vi "ROS_Publisher.vi"() -> ()   [LabVIEW 2016]
doc: "The ROS publisher bundles together several variables into a \"MasterMessage\" that is published on the ROS network. If there is an error in the ROS Write node the VI is exited."
uses:
  <userlib>/ROS for LabVIEW Software/ROS/Code/Console/Servers/ServerSubs/TopicDef.ctl
  <userlib>/ROS for LabVIEW Software/ROS/Code/SubVIs/_ROSDirection.ctl
  GlobalVI.vi
  <userlib>/ROS for LabVIEW Software/ROS/Code/_ROSDefinition.vi
panel:
  out "ROS Write ERR":errorcluster
  out "JSON string 2":string
  out "error out":errorcluster
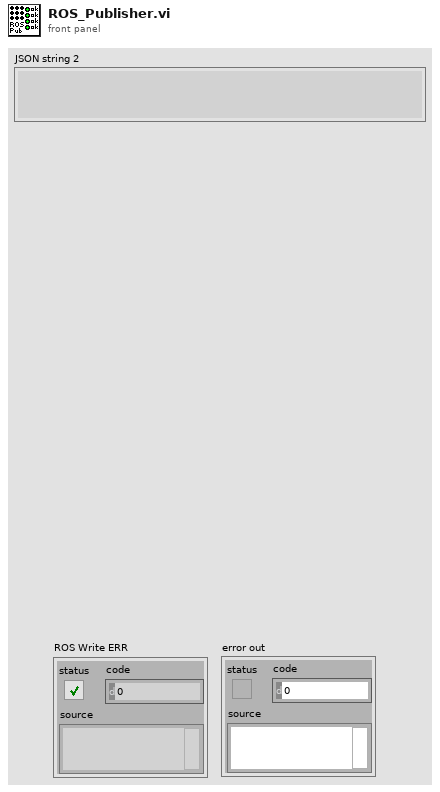
[diagram p1: front panel]
types:
  T1 = typedef "TopicDef.ctl" = cluster{"Topic":string, "Type":string, "Action":T2, "Update (ms)":u16, "queue size":u16}
  T2 = typedef "_ROSDirection.ctl" = enum16{"Node", "Publisher", "Subscriber", "ServiceClient", "ServiceProvider"}
  T3 = typedef "_ROSControl.ctl" = cluster{"topic port":u16, "Node":string, "topic":string, "type":string, "node port":u16, "error ":errorcluster, "Direction":T2, "Update (ms)":u16, "FIFO size":u16}
  T4 = cluster{"status":cluster{"liftStatus":bool, "lidarBackStatus":bool, "uwbStatus":bool, "lightStatus":bool}}
  T5 = cluster{"liftStatus":bool, "lidarBackStatus":bool, "uwbStatus":bool, "lightStatus":bool}
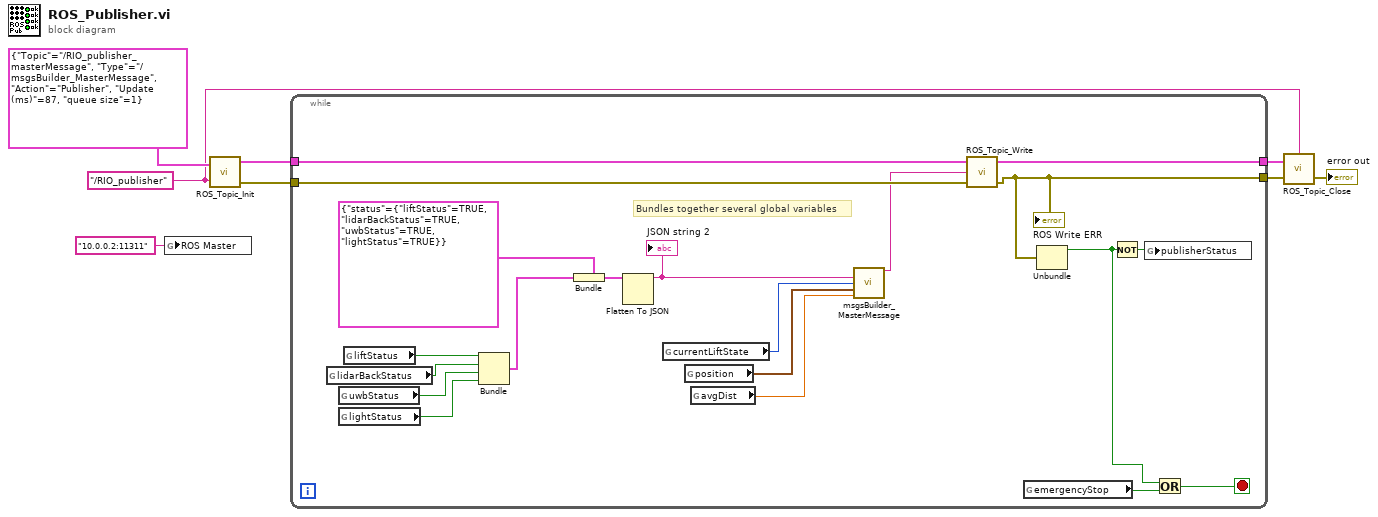
[diagram p0: block diagram]
diagram:
  w7 = "/RIO_publisher" ("node")
  n1 = global write "_ROSDefinition.vi" "ROS Master"("10.0.0.2:11311" ("ROS Master")) -> ()
  n2 = call <userlib>:"ROS_Topic_Init.vi"("Definitions"=T1 {"Topic"="/RIO_publisher_masterMessage", "Type"="/msgsBuilder_MasterMessage", "Action"=enum."Publisher", "Update (ms)"=87, "queue size"=1}, "node"=w7) -> ("ROS out"=w6:T3, "error out"=w1:errorcluster)  [unwired: 1 in]
  n3 = while {
    tunnel: w6 -> [w28]
    tunnel: [w27] -> w5
    tunnel: w1 -> [w26]
    tunnel: [w18] -> w4
    stop <- w16 stop-if-true
    # "Bundles together several global variables"
    n4 = global read "GlobalVI.vi" "lidarBackStatus"() -> (w23:bool)
    n5 = global read "GlobalVI.vi" "uwbStatus"() -> (w24:bool)
    n6 = global read "GlobalVI.vi" "lightStatus"() -> (w25:bool)
    n7 = global read "GlobalVI.vi" "liftStatus"() -> (w22:bool)
    n8 = Bundle("liftStatus"=w22, "lidarBackStatus"=w23, "uwbStatus"=w24, "lightStatus"=w25) -> (w20:T5)  [unwired: 1 in]
    n9 = Bundle(cluster=T4 {"status"={"liftStatus"=TRUE, "lidarBackStatus"=TRUE, "uwbStatus"=TRUE, "lightStatus"=TRUE}}, "status"=w20) -> (w19:T4)
    n10 = Flatten To JSON(anything=w19) -> (JSON string=w15:string)  [unwired: 2 in, 1 out]
    "JSON string 2" <- w15
    n11 = global read "GlobalVI.vi" "currentLiftState"() -> (w14:i32)
    n12 = global read "GlobalVI.vi" "position"() -> (w13:cluster{"x":dbl, "y":dbl, "z":dbl})
    n13 = global read "GlobalVI.vi" "avgDist"() -> (w12:sgl)
    n14 = call "msgsBuilder_MasterMessage.vi"("statusString"=w15, "liftState"=w14, "position"=w13, "avgDist"=w12) -> ("msg out"=w11:string)  [unwired: 11 in]
    n15 = call <userlib>:"ROS_Topic_Write.vi"("error in (no error)"=w26, "Msg in"=w11, "ROS in"=w28) -> ("error out"=w18:errorcluster, "ROS out"=w27:T3)  [unwired: 1 in]
    "ROS Write ERR" <- w18
    n16 = global read "GlobalVI.vi" "emergencyStop"() -> (w17:bool)
    n17 = Unbundle(w18) -> ("status"=w9:bool)  [unwired: 2 out]
    n18 = Not(x=w9) -> (.not. x?=w10:bool)
    n19 = global write "GlobalVI.vi" "publisherStatus"(w10) -> ()
    n20 = Or(x=w9, y=w17) -> (x .or. y?=w16:bool)
  }
  n21 = call <userlib>:"ROS_Topic_Close.vi"("error in"=w4, "ROS in"=w5, "node"=w7) -> ("error out"=→"error out":errorcluster)  [unwired: 1 in]
